vi "Read array type.vi"(8 "error in (no error)":errorcluster, 11 "JSON Array in":refnum<class "JSON Array.lvclass">) -> (0 "error out":errorcluster, 2 "datatype":T1, 3 "JSON Array out":refnum<class "JSON Array.lvclass">)   [LabVIEW 2017]
uses:
  JSON Array.lvclass
  C:/Users/tblair/Documents/JSON Parsing Experiments/JSON Data Classes/JSON Structured Type/JSON Structured Type.lvclass
  C:/Users/tblair/Documents/JSON Parsing Experiments/JSON Data Classes/JSON Datatype/JSON Datatype.lvclass
  JSON Types.ctl
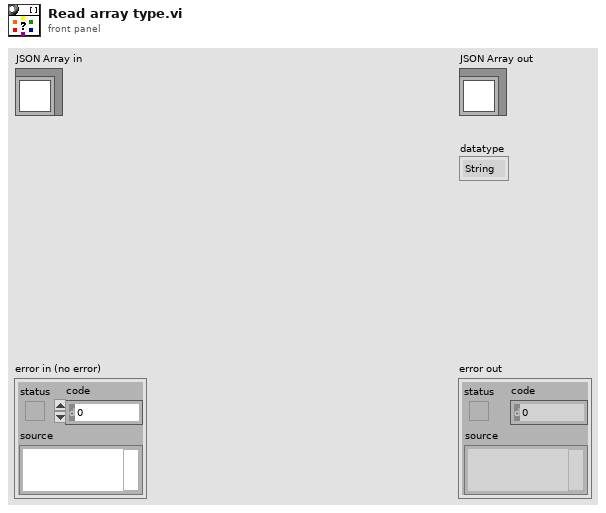
[diagram p1: front panel]
types:
  T1 = typedef "JSON Types.ctl" = enum16{"String", "Numeric", "Boolean", "NULL", "Object", "1D Array", "1D String", "1D Numeric", "1D Boolean"}
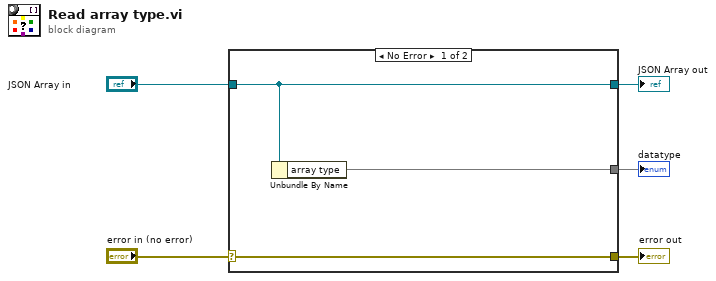
[diagram p0: block diagram]
diagram:
  n1 = case shown="No Error" "error in (no error)" {
    selector: "error in (no error)" -> [w8 w9]
    tunnel: [w8 w9] -> w4
    tunnel: [w7 w10] -> w2
    tunnel: "JSON Array in" -> [w7 w10]
    tunnel: [w6 _] -> w1
    frame No Error {
      n2 = Unbundle By Name(w7) -> ("array type"=w6)
    }
    frame Error {
    }
  }
  "error out" <- w4
  "JSON Array out" <- w2
  "datatype" <- w1
